vi "State Logic.vi"(0 "TLB' data in":refnum<class "{TMPL} TLB`.lvclass">, 1 "process state logic enable":bool, 5 "trigger queue in":refnum<queue>, 7 "action queue in":refnum<queue>, 11 "error in":errorcluster) -> (4 "TLB' data out":refnum<class "{TMPL} TLB`.lvclass">, 15 "error out":errorcluster)   [LabVIEW 2015, in "TLB` Template.lvlib" / "{TMPL} TLB`.lvclass"]
doc: "Control process for TLB' template.\n\n<B>Input Parameters</B>\n\n<B>TLB' data in</B> is the templates' private data.\n\n<B>process state logic enable</B> enable state logic change.\n\n<B>trigger queue in</B> is a reference to a queue. Use the Create Trigger Queue function to obtain a queue reference. \n\n<B>action queue in</B> is a reference to a queue. Use the Create Action Queue function to obtain a queue reference. \n\n<B>timeout (ms)</B> queue timeout.\n\n<B>error in</B> describes error conditions that occur before this node runs. This input provides standard error in functionality.\n\n<B>Output Parameters</B>\n\n<B>TLB' data out</B> is the templates' private data.\n\n<B>error out</B> contains error information. This output provides standard error out functionality."
uses:
  {TMPL} TLB`.lvclass
  Application Components/Trigger API/System Trigger Element.ctl
  Application Components/Trigger API/System Trigger.ctl
  Core Components/Actions/System Action Element.ctl
  {TMPL} TLB`.lvclass/{TMPL} TLB`.ctl
  State.ctl
  Core Components/Error Handler/TLB` Error Handler.lvclass/TLB` Error Handler.ctl
  Core Components/Error Handler/accessors/Get Action Causing Error.vi
  Core Components/Error Handler/accessors/Get Originating State.vi
  Core Components/Error Handler/accessors/Get Destination State.vi
  Core Components/Error Handler/accessors/Get Executed System Actions.vi
  Core Components/Error Handler/accessors/Get Remaing System Actions.vi
  Core Components/Error Handler/Core/actions/support/Error FLUSH-LOG-DIALOG.vi
  Core Components/Error Handler/Core/actions/support/Error DIALOG.vi
  Application Components/Trigger API/{TMPL} Trigger API.lvlib
  Core Components/Error Handler/TLB` Error Handler.lvclass
  Core Components/Actions/Actions.lvlib
  TLB` Template.lvlib
  Core Components/Error Handler/Core/actions/support/Error FLUSH-DIALOG.vi
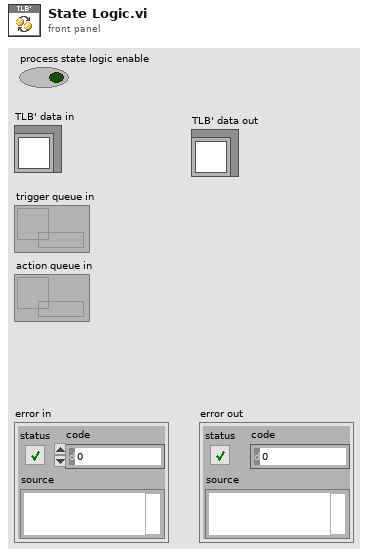
[diagram p1: front panel]
types:
  T1 = typedef "TLB` Template.lvlib/{TMPL} TLB`.lvclass/State.ctl" = enum16{"<Startup>", "Idle", "<Shutdown>", "<Error>"}
  T2 = typedef "TLB` Template.lvlib/{TMPL} Trigger API.lvlib/System Trigger.ctl" = enum16{"<None>", "Connect", "Start Acquisition", "Stop Acquisition", "Disconnect", "<Return to Safe State Actions>", "<Cache User Parameters>", "<Close Application>", "<Error>"}
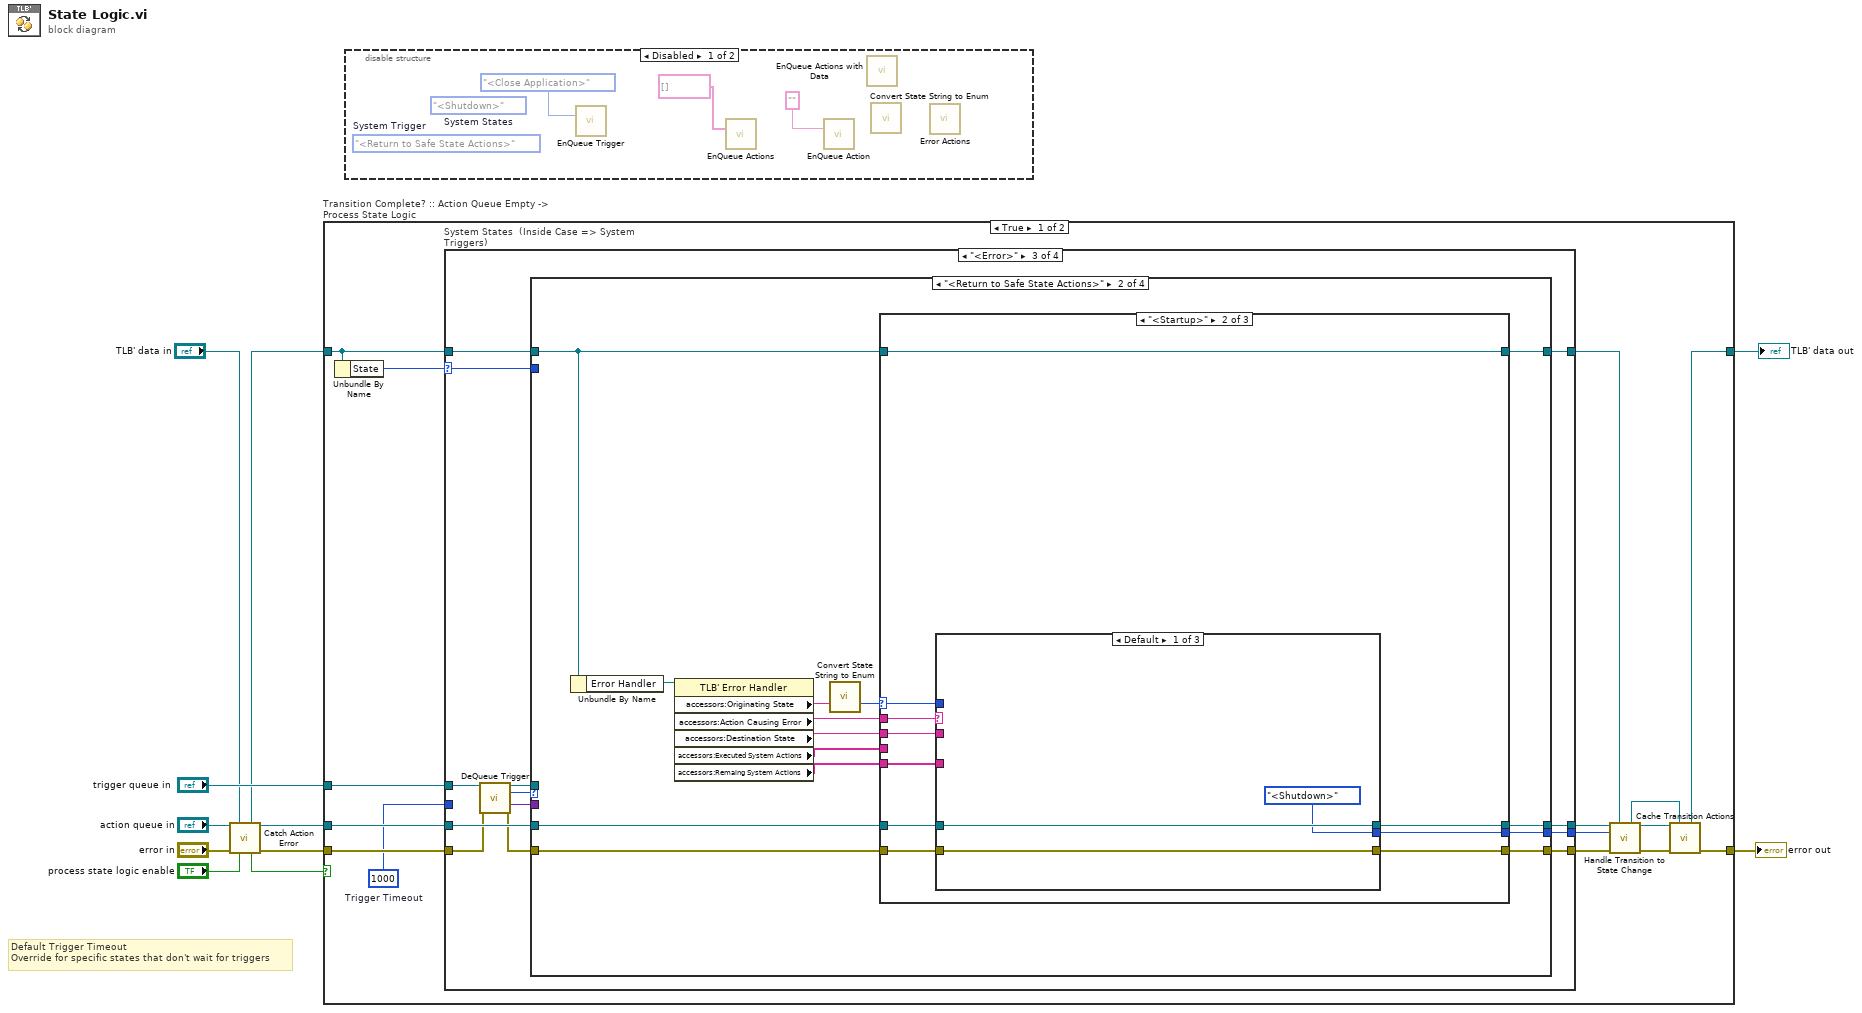
[diagram p0: block diagram]
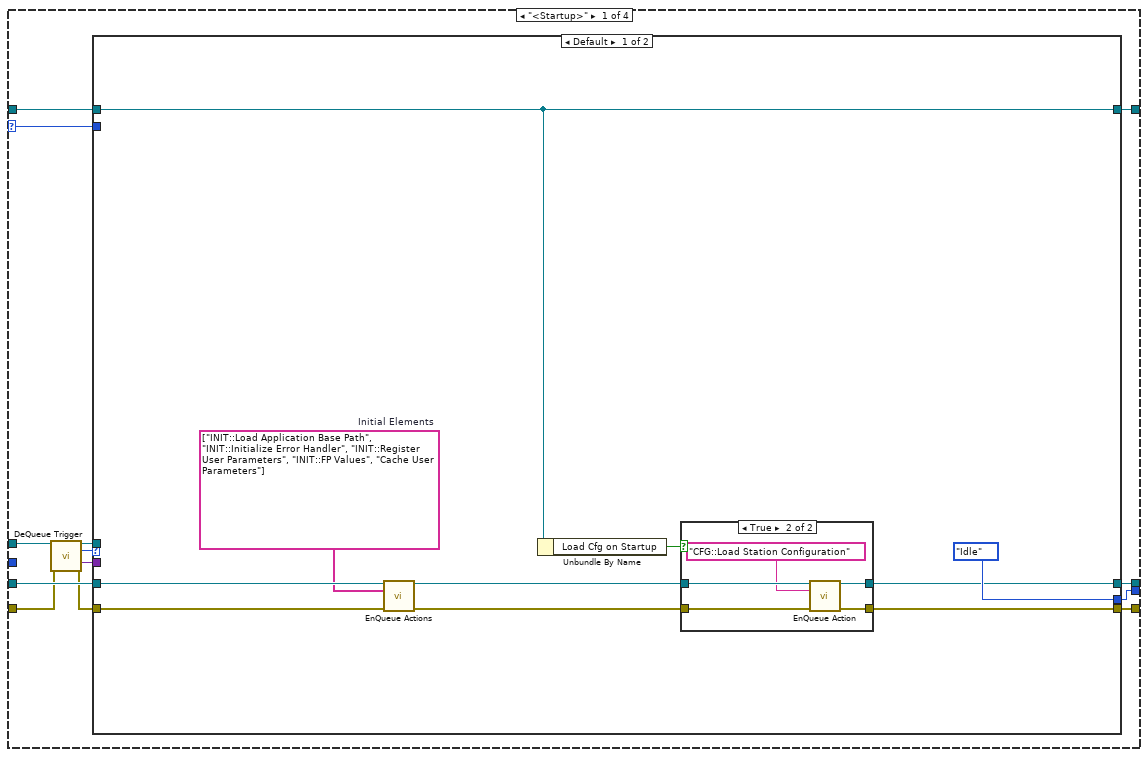
[diagram p3: hidden frame]
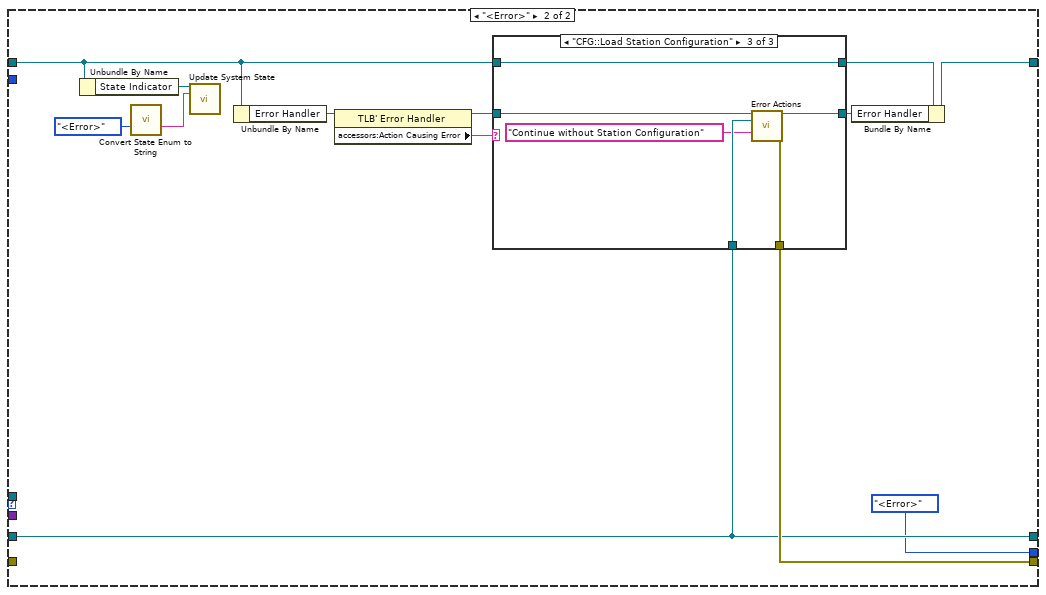
[diagram p5: hidden frame]
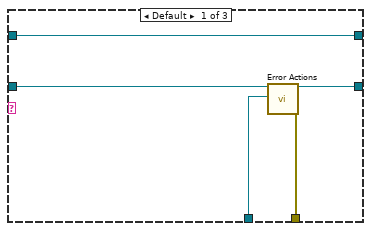
[diagram p6: hidden frame]
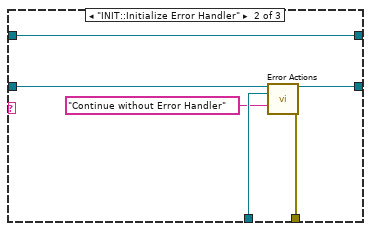
[diagram p7: hidden frame]
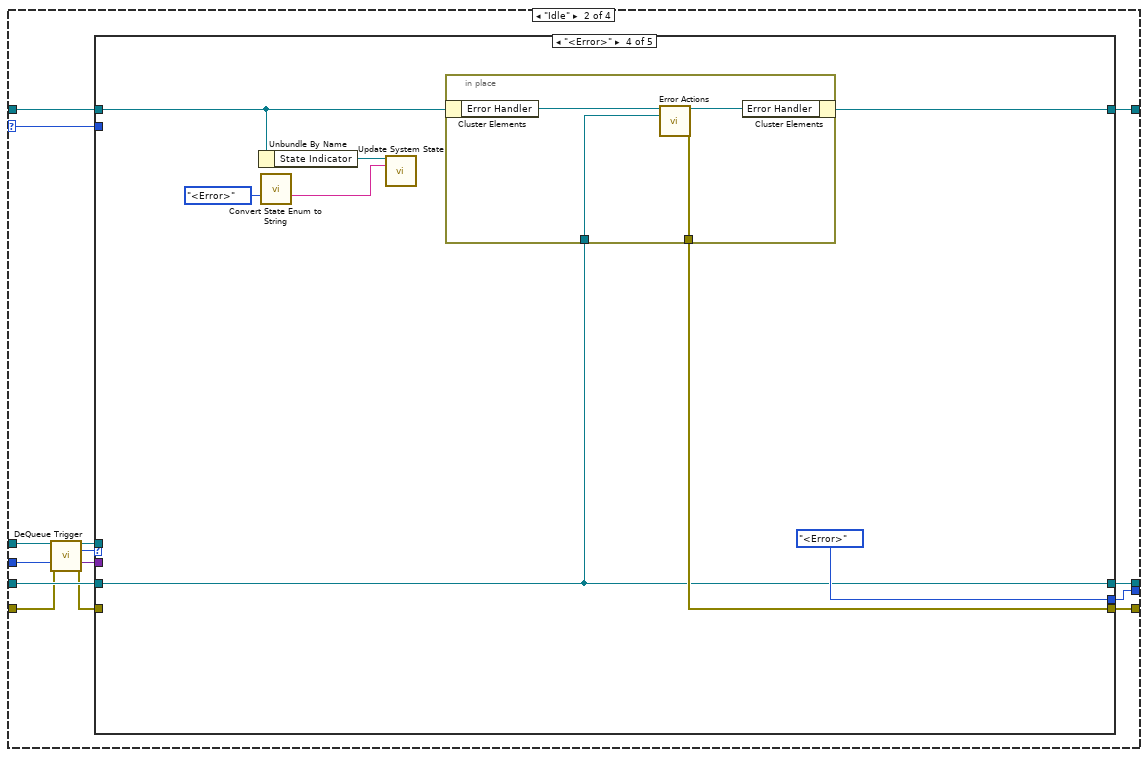
[diagram p8: hidden frame]
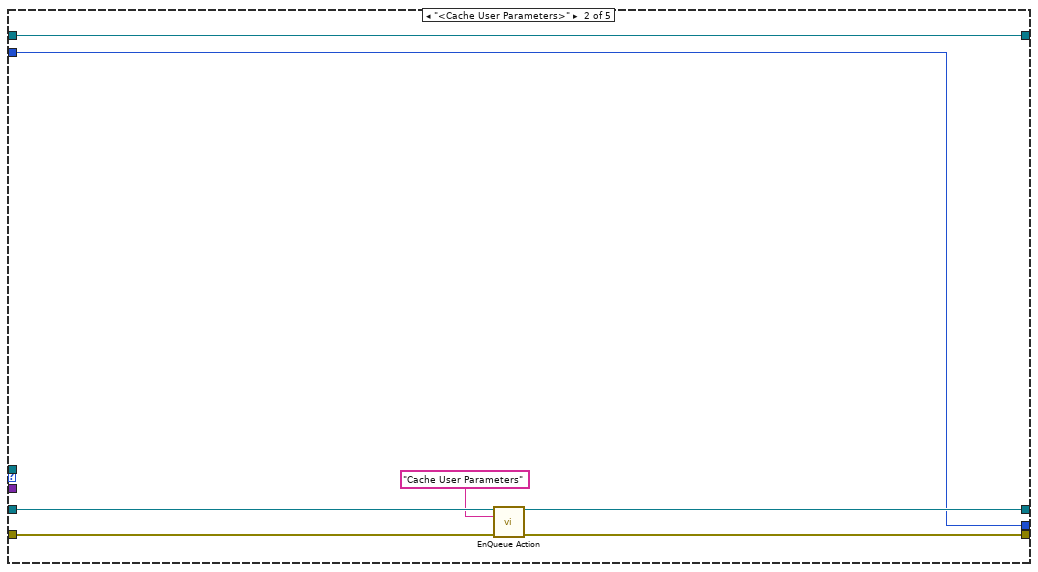
[diagram p10: hidden frame]
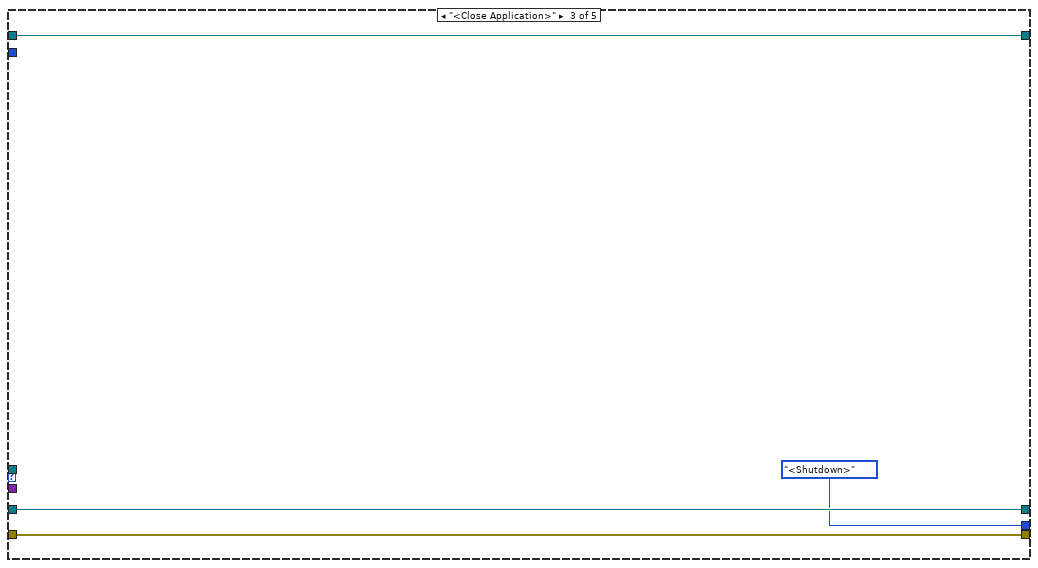
[diagram p11: hidden frame]
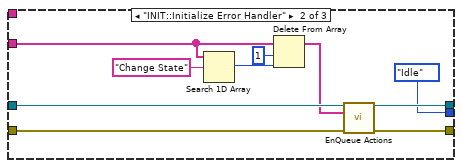
[diagram p15: hidden frame]
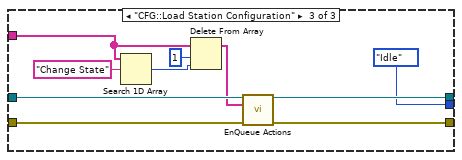
[diagram p16: hidden frame]
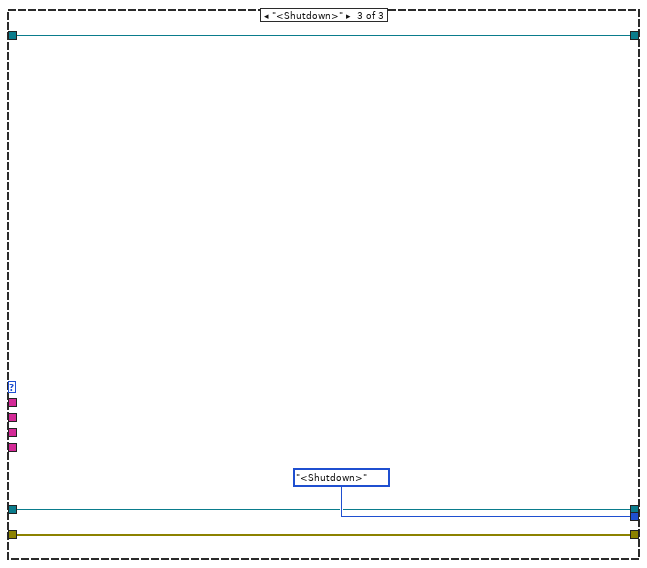
[diagram p17: hidden frame]
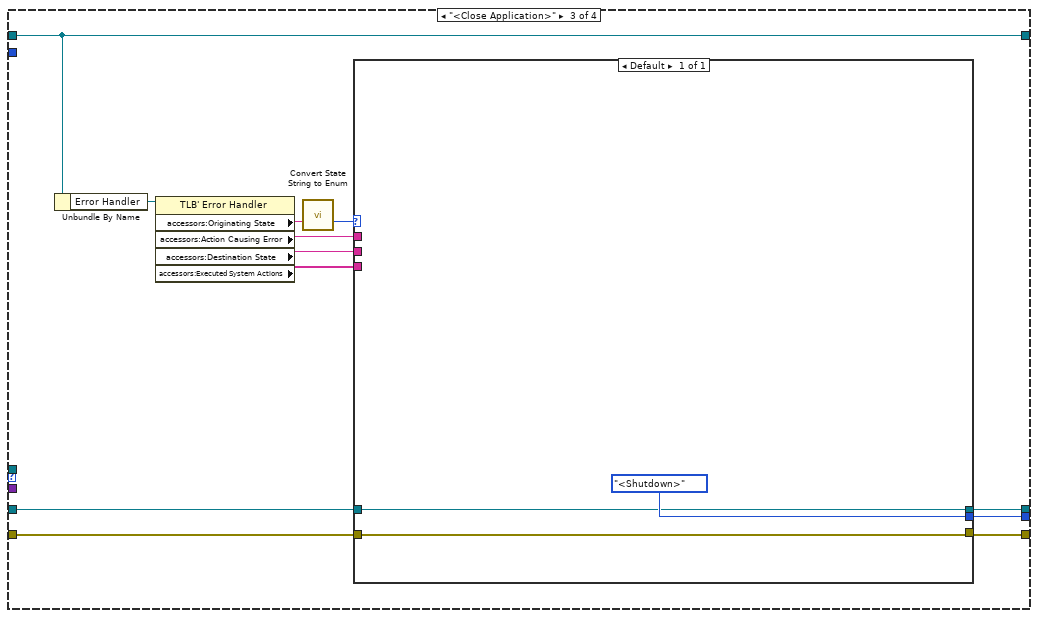
[diagram p18: hidden frame]
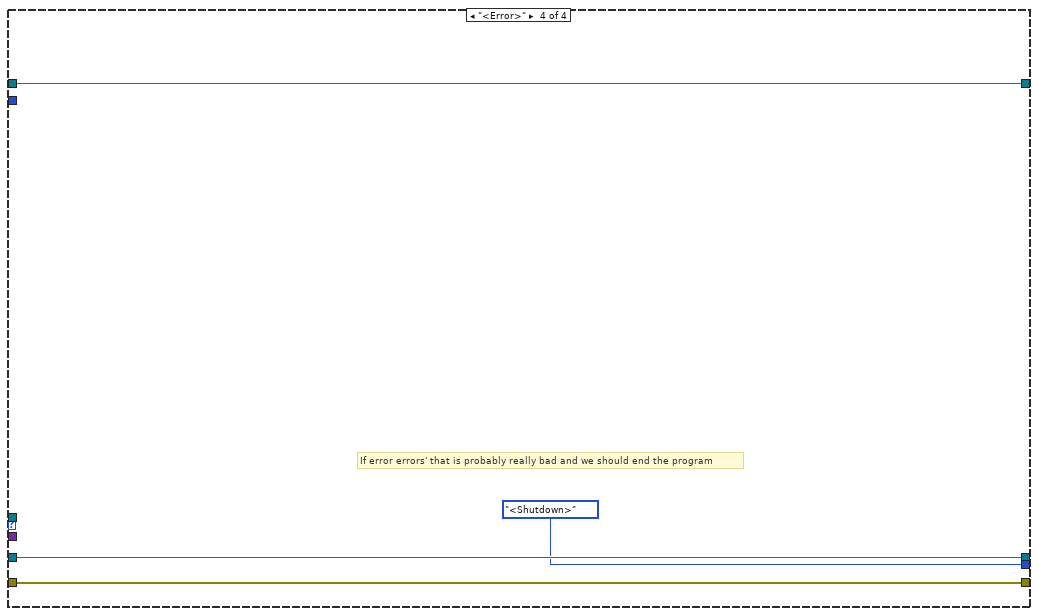
[diagram p19: hidden frame]
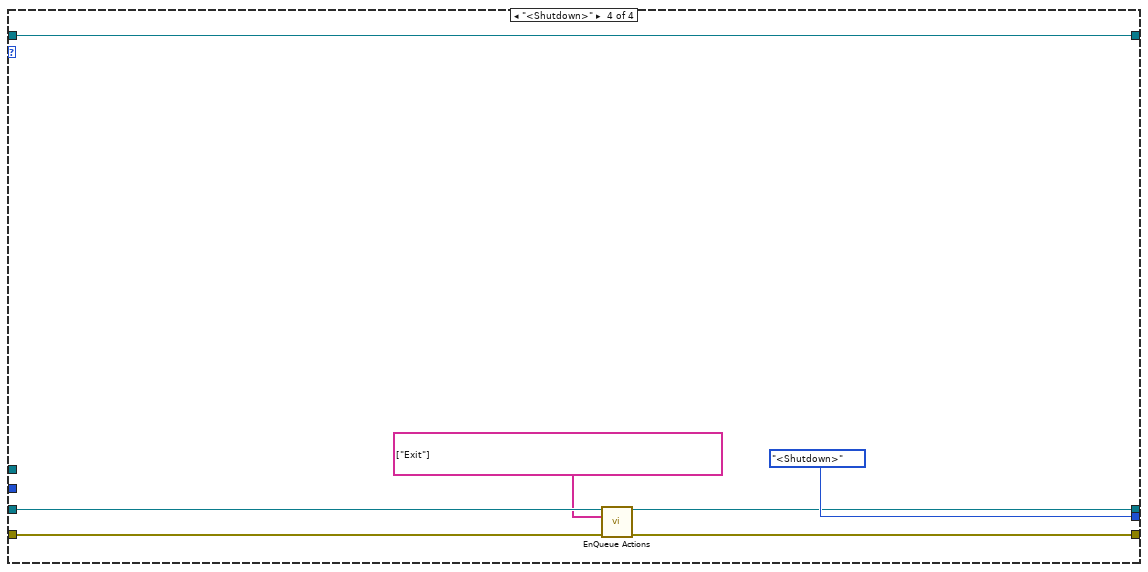
[diagram p20: hidden frame]
diagram:
  # "Default Trigger Timeout\nOverride for specific states that don't wait for triggers"
  n1 = call "Catch Action Error.vi"("action queue in"="action queue in", "TLB' Template in"="TLB' data in", "error in (no error)"="error in", "process state logic enable in"="process state logic enable") -> ("TLB' Template out"=w6:refnum<class "{TMPL} TLB`.lvclass">, "action queue in"=w2:refnum<queue>, "process state logic enable out"=w4:bool, "error out"=w7:errorcluster)  [unwired: 8 in]
  n2 = case "Transition Complete? :: Action Queue Empty -> Process State Logic" shown="True" w4 {
    tunnel: [w17 w230] -> w10
    tunnel: w6 -> [w22 w230]
    tunnel: w7 -> [w26 w231]
    tunnel: w2 -> [w25 _]
    tunnel: [w20 w231] -> w11
    tunnel: "trigger queue in" -> [w24 _]
    frame True {
      w18 = 1000  # Trigger Timeout
      n3 = Unbundle By Name(w22) -> ("State"=w19:T1)
      n4 = case "System States  (Inside Case => System Triggers)" shown="\"<Error>\"" w19 {
        selector: w19 -> [w27 w89 w139 _]
        tunnel: [w33 w94 w137 w228] -> w15
        tunnel: w22 -> [w34 w95 w138 w228]
        tunnel: w26 -> [w32 w93 w136 w227]
        tunnel: w25 -> [w38 w99 w140 w226]
        tunnel: [w37 w98 w143 w224] -> w23
        tunnel: w24 -> [w39 w100 w144 _]
        tunnel: [w36 w97 w142 w225] -> w16
        tunnel: [w35 w96 w141 State."<Shutdown>" ("State")] -> w12
        tunnel: w18 -> [_ w88 _ _]
        frame "<Startup>" {
          n5 = call "DeQueue Trigger.vi"("trigger queue in"=w39, "error in"=w32) -> ("trigger queue out"=w28:refnum<queue>, "system trigger"=w30:T2, "trigger data"=w29:variant, "error out"=w31:errorcluster)  [unwired: 10 in]
          n6 = case shown="Default" w30 {
            tunnel: w31 -> [w46 _]
            tunnel: w38 -> [w48 w67]
            tunnel: [w43 w68] -> w37
            tunnel: [w41 w67] -> w36
            tunnel: w29 -> [_ _]
            tunnel: [State."Idle" ("State") State."<Error>" ("State")] -> w35
            tunnel: w34 -> [w44 w58]
            tunnel: [w44 w69] -> w33
            tunnel: w28 -> [_ _]
            tunnel: w27 -> [_ _]
            frame Default {
              w47 = string[] ["INIT::Load Application Base Path", "INIT::Initialize Error Handler", "INIT::Register User Parameters", "INIT::FP Values", "Cache User Parameters"]  # Initial Elements
              n7 = call "EnQueue Actions.vi"("action queue in"=w48, "actions"=w47, "error in"=w46) -> ("action queue out"=w42:refnum<queue>, "error out"=w45:errorcluster)  [unwired: 11 in]
              n8 = Unbundle By Name(w44) -> ("Load Cfg on Startup"=w40:bool)
              n9 = case shown="True" w40 {
                tunnel: w45 -> [w50 w56]
                tunnel: [w50 w55] -> w43
                tunnel: w42 -> [w51 w54]
                tunnel: [w51 w53] -> w41
                frame False {
                }
                frame True {
                  n10 = call "EnQueue Action.vi"("action queue in"=w54, "action"="CFG::Load Station Configuration", "error in"=w56) -> ("action queue out"=w53:refnum<queue>, "error out"=w55:errorcluster)  [unwired: 11 in]
                }
              }
            }
            frame "<Error>" {
              n11 = Unbundle By Name(w58) -> ("State Indicator"=w62:refnum<user-event>)
              n12 = call "Convert State Enum to String.vi"("state in"=State."<Error>") -> ("state out"=w61:string)  [unwired: 13 in, 1 out]
              n13 = call "Update System State.vi"("State Indicator"=w62, "system state message"=w61) -> ()  [unwired: 13 in, 1 out]
              n14 = Unbundle By Name(w58) -> ("Error Handler"=w64:refnum<class "TLB` Error Handler.lvclass">)
              n15 = property class="TLB' Error Handler"(reference=w64) -> (reference out=w63:refnum<class "TLB` Error Handler.lvclass">, "accessors:Action Causing Error"=w60:string)  [unwired: 1 in, 1 out]
              n16 = case shown="\"CFG::Load Station Configuration\"" w60 {
                tunnel: [w72 w80 w86] -> w68
                tunnel: w67 -> [w71 w79 w85]
                tunnel: [w73 w78 w84] -> w65
                tunnel: w63 -> [w74 w77 w83]
                tunnel: w58 -> [w70 w75 w81]
                tunnel: [w70 w75 w81] -> w57
                frame Default {
                  n17 = call-poly "Error Actions.vi"("Error Handler in"=w74, "action queue in"=w71) -> ("Error Handler out"=w73:refnum<class "TLB` Error Handler.lvclass">, "error out"=w72:errorcluster)  [unwired: 12 in]
                }
                frame "INIT::Initialize Error Handler" {
                  n18 = call-poly "Error Actions.vi"("Error Handler in"=w77, "action queue in"=w79, "error button text (Return to Safe State)"="Continue without Error Handler") -> ("Error Handler out"=w78:refnum<class "TLB` Error Handler.lvclass">, "error out"=w80:errorcluster)  [unwired: 11 in]
                }
                frame "CFG::Load Station Configuration" {
                  n19 = call-poly "Error Actions.vi"("Error Handler in"=w83, "action queue in"=w85, "error button text (Return to Safe State)"="Continue without Station Configuration") -> ("Error Handler out"=w84:refnum<class "TLB` Error Handler.lvclass">, "error out"=w86:errorcluster)  [unwired: 11 in]
                }
              }
              n20 = Bundle By Name(cluster=w57, "Error Handler"=w65) -> (w69:refnum<class "{TMPL} TLB`.lvclass">)
            }
          }
        }
        frame "Idle" {
          n21 = call "DeQueue Trigger.vi"("trigger queue in"=w100, "timeout, ms (0)"=w88, "error in"=w93) -> ("trigger queue out"=w87:refnum<queue>, "system trigger"=w91:T2, "trigger data"=w90:variant, "error out"=w92:errorcluster)  [unwired: 9 in]
          n22 = case shown="\"<Error>\"" w91 {
            tunnel: w92 -> [w103 w111 w114 _ w130]
            tunnel: w99 -> [w104 w108 w115 w119 w131]
            tunnel: [w103 w109 w114 w121 w130] -> w98
            tunnel: [w104 w107 w115 w119 w131] -> w97
            tunnel: w90 -> [_ _ _ _ _]
            tunnel: w95 -> [w102 w110 w113 w118 w129]
            tunnel: [w101 w105 State."<Shutdown>" ("State") State."<Error>" ("State") w128] -> w96
            tunnel: [w102 w110 w113 w120 w129] -> w94
            tunnel: w89 -> [w101 w105 _ _ w128]
            tunnel: w87 -> [_ _ _ _ _]
            frame "<None>" {
            }
            frame "<Cache User Parameters>" {
              n23 = call "EnQueue Action.vi"("action queue in"=w108, "action"="Cache User Parameters", "error in"=w111) -> ("action queue out"=w107:refnum<queue>, "error out"=w109:errorcluster)  [unwired: 11 in]
            }
            frame "<Close Application>" {
            }
            frame "<Error>" {
              n24 = Unbundle By Name(w118) -> ("State Indicator"=w122:refnum<user-event>)
              n25 = call "Convert State Enum to String.vi"("state in"=State."<Error>") -> ("state out"=w116:string)  [unwired: 13 in, 1 out]
              n26 = call "Update System State.vi"("State Indicator"=w122, "system state message"=w116) -> ()  [unwired: 13 in, 1 out]
              n27 = in-place {
                in-place-border: [w125] -> w121
                in-place-border: w119 -> [w124]
                n28 = in-place-cluster #1(w118) -> ("Error Handler"=w127:refnum<class "TLB` Error Handler.lvclass">)
                n29 = call-poly "Error Actions.vi"("Error Handler in"=w127, "action queue in"=w124) -> ("Error Handler out"=w126:refnum<class "TLB` Error Handler.lvclass">, "error out"=w125:errorcluster)  [unwired: 12 in]
                n30 = in-place-cluster #1("Error Handler"=w126) -> (w120:refnum<class "{TMPL} TLB`.lvclass">)
              }
            }
            frame Default {
            }
          }
        }
        frame "<Error>" {
          n31 = call "DeQueue Trigger.vi"("trigger queue in"=w144, "error in"=w136) -> ("trigger queue out"=w135:refnum<queue>, "system trigger"=w134:T2, "trigger data"=w132:variant, "error out"=w133:errorcluster)  [unwired: 10 in]
          n32 = case shown="\"<Return to Safe State Actions>\"" w134 {
            tunnel: w138 -> [w146 w149 w204 w220]
            tunnel: [w147 w159 w213 w219] -> w143
            tunnel: w133 -> [w147 w161 w214 w219]
            tunnel: w140 -> [w148 w162 w215 w222]
            tunnel: [w148 w160 w210 w222] -> w142
            tunnel: [w145 w158 w212 State."<Shutdown>" ("State")] -> w141
            tunnel: w135 -> [_ _ _ _]
            tunnel: w139 -> [w145 _ _ _]
            tunnel: w132 -> [_ _ _ _]
            tunnel: [w146 w157 w204 w220] -> w137
            frame Default {
            }
            frame "<Return to Safe State Actions>" {
              n33 = Unbundle By Name(w149) -> ("Error Handler"=w156:refnum<class "TLB` Error Handler.lvclass">)
              n34 = property class="TLB' Error Handler"(reference=w156) -> ("accessors:Originating State"=w151:string, "accessors:Action Causing Error"=w155:string, "accessors:Destination State"=w154:string, "accessors:Executed System Actions"=w153:string[], "accessors:Remaing System Actions"=w150:string[])  [unwired: 1 in, 2 out]
              n35 = call "Convert State String to Enum.vi"("state in"=w151) -> ("state out"=w152:T1)  [unwired: 13 in, 1 out]
              n36 = case shown="\"<Startup>\"" w152 {
                selector: w152 -> [w163 w168 _]
                tunnel: w162 -> [w166 w174 w201]
                tunnel: w161 -> [w164 w175 w200]
                tunnel: [w164 w173 w200] -> w159
                tunnel: [w166 w172 w201] -> w160
                tunnel: [w163 w171 State."<Shutdown>" ("State")] -> w158
                tunnel: w149 -> [w165 w176 w203]
                tunnel: [w165 w176 w203] -> w157
                tunnel: w155 -> [_ w170 _]
                tunnel: w154 -> [_ w167 _]
                tunnel: w153 -> [_ _ _]
                tunnel: w150 -> [_ w169 _]
                frame Default {
                }
                frame "<Startup>" {
                  n37 = case shown="Default" w170 {
                    tunnel: w175 -> [w178 w188 w198]
                    tunnel: w174 -> [w179 w189 w199]
                    tunnel: [w178 w187 w197] -> w173
                    tunnel: [w179 w186 w196] -> w172
                    tunnel: [State."<Shutdown>" ("State") State."Idle" ("state out") State."Idle" ("state out")] -> w171
                    tunnel: w169 -> [_ w185 w195]
                    tunnel: w168 -> [_ _ _]
                    tunnel: w167 -> [_ _ _]
                    frame Default {
                    }
                    frame "INIT::Initialize Error Handler" {
                      n38 = Search 1D Array(1D array=w185, element="Change State") -> (index of element=w183:i32)  [unwired: 1 in]
                      n39 = Delete From Array(array=w185, length=1, index=w183) -> (array with subset deleted=w184:string[])  [unwired: 1 out]
                      n40 = call "EnQueue Actions.vi"("action queue in"=w189, "actions"=w184, "error in"=w188) -> ("action queue out"=w186:refnum<queue>, "error out"=w187:errorcluster)  [unwired: 11 in]
                    }
                    frame "CFG::Load Station Configuration" {
                      n41 = Search 1D Array(1D array=w195, element="Change State") -> (index of element=w193:i32)  [unwired: 1 in]
                      n42 = Delete From Array(array=w195, length=1, index=w193) -> (array with subset deleted=w194:string[])  [unwired: 1 out]
                      n43 = call "EnQueue Actions.vi"("action queue in"=w199, "actions"=w194, "error in"=w198) -> ("action queue out"=w196:refnum<queue>, "error out"=w197:errorcluster)  [unwired: 11 in]
                    }
                  }
                }
                frame "<Shutdown>" {
                }
              }
            }
            frame "<Close Application>" {
              n44 = Unbundle By Name(w204) -> ("Error Handler"=w211:refnum<class "TLB` Error Handler.lvclass">)
              n45 = property class="TLB' Error Handler"(reference=w211) -> ("accessors:Originating State"=w209:string, "accessors:Action Causing Error"=w205:string, "accessors:Destination State"=w206:string, "accessors:Executed System Actions"=w207:string[])  [unwired: 1 in, 2 out]
              n46 = call "Convert State String to Enum.vi"("state in"=w209) -> ("state out"=w208:T1)  [unwired: 13 in, 1 out]
              n47 = case shown="Default" w208 {
                tunnel: w215 -> [w217]
                tunnel: w214 -> [w216]
                tunnel: [w216] -> w213
                tunnel: [w217] -> w210
                tunnel: [State."<Shutdown>" ("State")] -> w212
                tunnel: w205 -> [_]
                tunnel: w206 -> [_]
                tunnel: w207 -> [_]
                frame Default {
                }
              }
            }
            frame "<Error>" {
              # "If error errors' that is probably really bad and we should end the program"
            }
          }
        }
        frame "<Shutdown>" {
          n48 = call "EnQueue Actions.vi"("action queue in"=w226, "actions"=string[] ["Exit"], "error in"=w227) -> ("action queue out"=w225:refnum<queue>, "error out"=w224:errorcluster)  [unwired: 11 in]
        }
      }
      n49 = call "Handle Transition to State Change.vi"("action queue in"=w16, "TLB' Template in"=w15, "Destination State"=w12, "error in (no error)"=w23) -> ("TLB' Template out"=w14:refnum<class "{TMPL} TLB`.lvclass">, "action queue in"=w13:refnum<queue>, "error out"=w21:errorcluster)  [unwired: 9 in]
      n50 = call "Cache Transition Actions.vi"("action queue in"=w13, "TLB' Template in"=w14, "error in (no error)"=w21) -> ("TLB' Template out"=w17:refnum<class "{TMPL} TLB`.lvclass">, "error out"=w20:errorcluster)  [unwired: 11 in]
    }
    frame False {
    }
  }
  "error out" <- w11
  "TLB' data out" <- w10
  n51 = disable-structure shown="Disabled" {
    frame Disabled {
      (unwired) System_Trigger."<Return to Safe State Actions>"  # System Trigger
      (unwired) State."<Shutdown>"  # System States
      n52 = call "EnQueue Trigger.vi"("system trigger"=System_Trigger."<Close Application>" ("System Trigger")) -> ()  [unwired: 13 in, 2 out]
      n53 = call "EnQueue Actions.vi"("actions"=string[] [] ("message names")) -> ()  [unwired: 13 in, 2 out]
      n54 = call "EnQueue Action.vi"("action"="" ("Message Name")) -> ()  [unwired: 13 in, 2 out]
      n55 = call "EnQueue Actions with Data.vi"() -> ()  [unwired: 14 in, 2 out]
      n56 = call "Convert State String to Enum.vi"() -> ()  [unwired: 14 in, 2 out]
      n57 = call-poly "Error Actions.vi"() -> ()  [unwired: 14 in, 2 out]
    }
    frame Enabled {
    }
  }
